vi "Failure Message.vi"() -> ()   [LabVIEW 2017, in "Assertions.Tests.lvlib" / "Assert String Not Ends With.lvlib"]
uses:
  Assert String Not Ends With.lvlib
  src/Transparent Assertions/Assertions/Assertions.lvlib
panel:
  out "error out":errorcluster
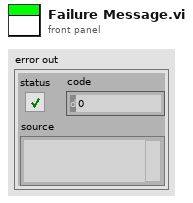
[diagram p1: front panel]
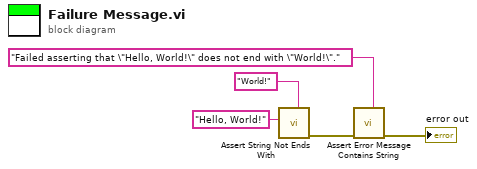
[diagram p0: block diagram]
diagram:
  n1 = call "Assert String Not Ends With.vi"("Suffix"="World!", "String"="Hello, World!") -> ("error out"=w5:errorcluster)  [unwired: 9 in]
  n2 = call "Assert Error Message Contains String.vi"("Expected"="Failed asserting that \"Hello, World!\" does not end with \"World!\".", "error in (no error)"=w5) -> ("error out"=→"error out":errorcluster)  [unwired: 9 in]
